vi "_Update Oscillators.vi"(4 "Pole In":bool[](array[boolean]), 5 "UpdateInput (F)":bool, 6 "ADC Array":i32[](array[numeric]), 7 "ADC Table":T1[](array[typedef]), 8 "Pole Swap (T)":bool=TRUE, 9 "Update (T)":bool=TRUE, 10 "Mode(pos)":bool=TRUE, 11 "Oscillator Settings":refnum<vi>) -> (1 "Q1RF Frequency":dbl, 2 "Instrument":string[](array[string]), 3 "Pole":bool[](array[boolean]))   [LabVIEW 2018]
uses:
  Type/_RT Configuration 2.ctl
  Type/_RT Command.ctl
  Configuration/_Global Configuration.vi
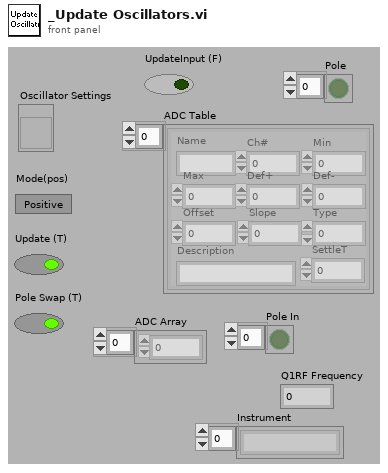
[diagram p1: front panel]
types:
  T1 = typedef "_RT Configuration 2.ctl" = cluster{"Name":string, "Ch#":u8, "Min":dbl, "Max":dbl, "Def+":dbl, "Def-":dbl, "Offset":dbl, "Slope":dbl, "Type":u8, "Description":string, "SettleT":dbl}
  T2 = typedef "_RT Instrument 2.ctl" = cluster{"Table":T1[], "Instrument":string[]}
  T3 = typedef "_RT Command.ctl" = enum16{"xml Start Run", "xml Start Actual Run", "xml Stop Run", "xml Runtime Update", "xml Get Status", "xml Get Table", "xml Set Table", "xml Get Configuration", "xml System Status", "xml Set LC Input Logic", "xml Get Data", "xml Get Info", "Start", "StartActualRun", "Stop", "Runtime Update", "Get Data", "Get Info", "Get Status", "Get Param", "Get Config", "Get Table", "Read ADC", "Set Oscillator", "Update Config", "Update Table", "Set All Pol", "Set Pol and DC", "Set Max Mass", "Toggle RP", "Toggle EL", "Set PIC", "Initialize Turbo", "Send Turbo Comm", "Close Turbo", "P1", "P2", "P3", "Send Serial", "Set LC Out", "Get LC In", "Read VAC", "Test Table", "Toggle Power", "Get Startup", "Set Startup", "Get ADC Table", "Set ADC Table", "Get Brief Status", "Get Detail Status", "Auxiliary Update", "Set CC Logics", "Test Channel", "Set CC Input Logics", "Ignore Error", "invalid"}
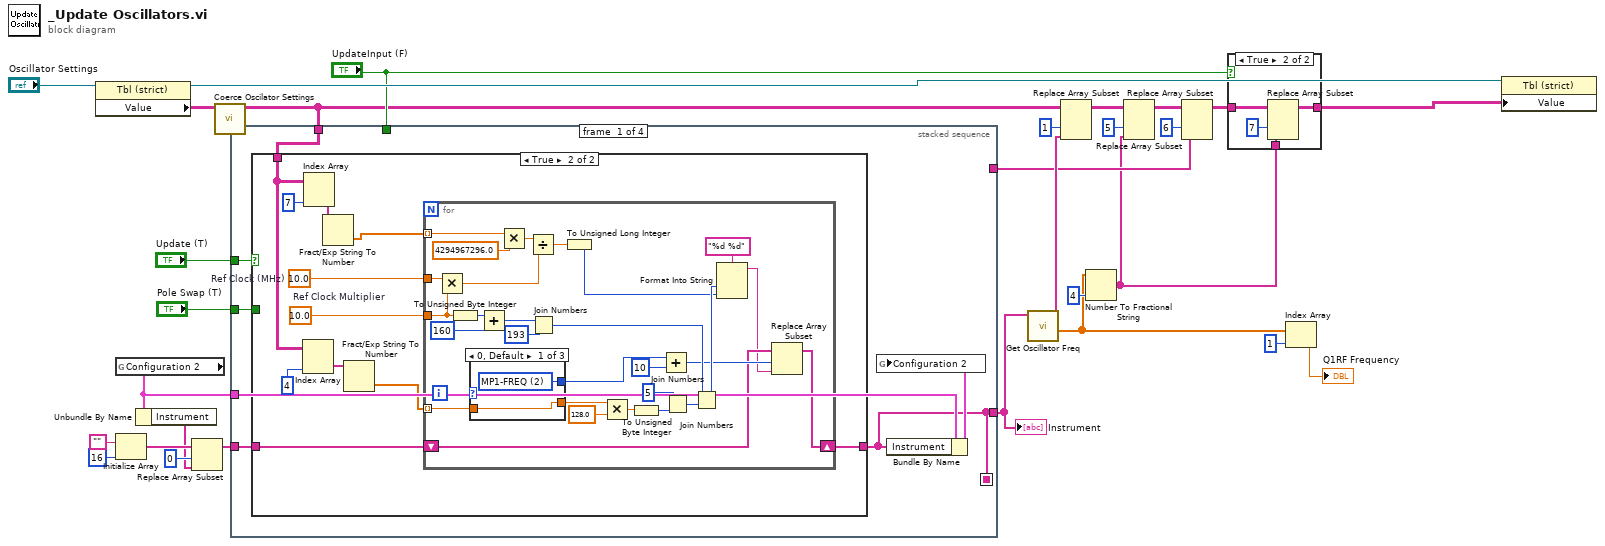
[diagram p0: block diagram]
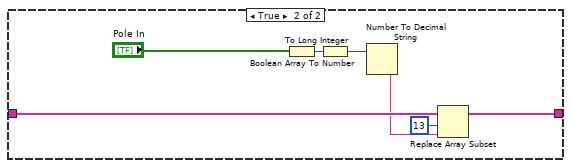
[diagram p4: hidden frame]
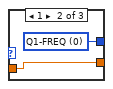
[diagram p5: hidden frame]
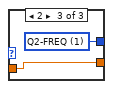
[diagram p6: hidden frame]
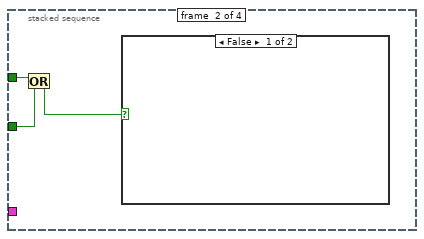
[diagram p7: hidden frame]
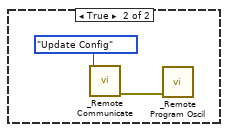
[diagram p8: hidden frame]
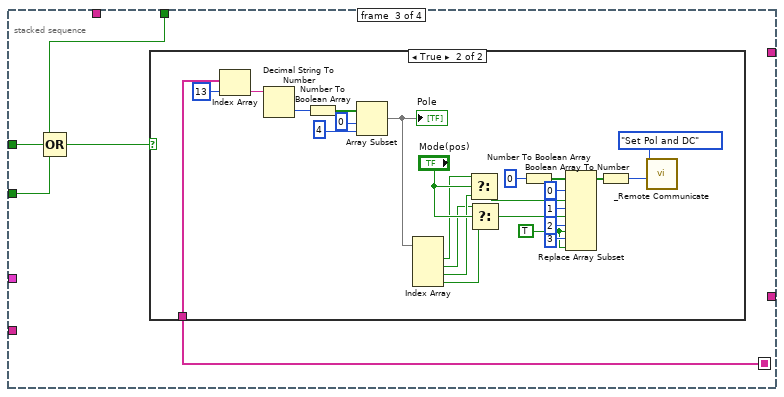
[diagram p9: hidden frame]
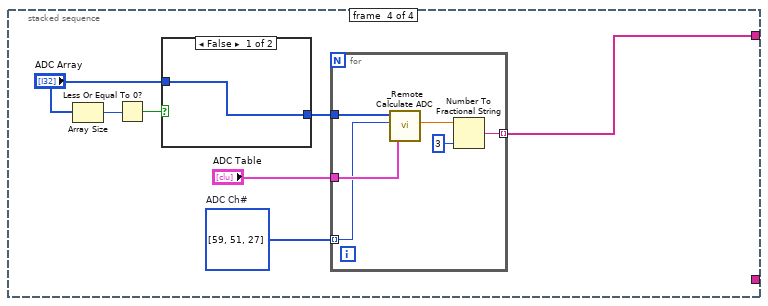
[diagram p11: hidden frame]
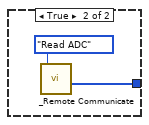
[diagram p12: hidden frame]
diagram:
  n1 = property class="Tbl (strict)"(reference="Oscillator Settings") -> (reference out=w21:refnum<vi>, "Value"=w14:string[][])  [unwired: 1 in, 1 out]
  n2 = global read "_Global Configuration.vi" "Configuration 2"() -> (w22:T2)
  n3 = Initialize Array("", 16 ("dimension size")) -> (w26:string[])
  n4 = Unbundle By Name(w22) -> ("Instrument"=w24:string[])
  n5 = Replace Array Subset(array=w26, new element=w24, index=0) -> (w23:string[])
  n6 = call "Coerce Oscilator Settings.vi"("Oscillator Settings in"=w14) -> ("Oscillator Settings out"=w4:string[][])  [unwired: 10 in]
  n7 = stacked-sequence {
    seq-local: [w30 _ _ _] -> [_ _ w103 _]
    tunnel: w4 -> [w36 _ _ _]
    tunnel: w23 -> [w35 _ _ _]
    tunnel: w22 -> [w33 _ _ _]
    tunnel: [w30 _ _ _] -> w16
    tunnel: "Update (T)" -> [w32 w96 w101 _]
    tunnel: "Pole Swap (T)" -> [w31 w95 w100 _]
    tunnel: [_ _ _ w132] -> w8
    tunnel: "UpdateInput (F)" -> [_ _ w102 _]
    frame #0 {
      n8 = case shown="True" w32 {
        tunnel: w36 -> [_ w51]
        tunnel: w35 -> [w39 w53]
        tunnel: [w37 w52] -> w30
        tunnel: w31 -> [w38 _]
        frame False {
          n9 = case shown="False" w38 {
            tunnel: w39 -> [w40 w45]
            tunnel: [w40 w44] -> w37
            frame False {
            }
            frame True {
              n10 = Boolean Array To Number(Boolean array="Pole In") -> (number=w46:u32)
              n11 = To Long Integer(number=w46) -> (32bit integer=w47:i32)
              n12 = Number To Decimal String(number=w47) -> (decimal integer string=w43:string)  [unwired: 1 out]
              n13 = Replace Array Subset(array=w45, new element=w43, index=13) -> (w44:string[])
            }
          }
        }
        frame True {
          w55 = 10.0  # Ref Clock Multiplier
          w56 = 10.0  # Ref Clock (MHz)
          n14 = Index Array(array=w51, index (col)=4 ("disabled index (col)")) -> (element=w50:string[])  [unwired: 1 in]
          n15 = Index Array(array=w51, index (col)=7 ("disabled index (col)")) -> (element=w57:string[])  [unwired: 1 in]
          n16 = Fract/Exp String To Number(string=w57) -> (number=w54:dbl[])  [unwired: 4 out]
          n17 = Fract/Exp String To Number(string=w50) -> (number=w48:dbl[])  [unwired: 4 out]
          n18 = for {
            tunnel: w56 -> [w83]
            tunnel: w55 -> [w80]
            tunnel: w54 -> [w61] mode=indexing
            shift-right: [w62] -> w52
            shift-left: w53 -> [w64]
            tunnel: w48 -> [w59] mode=indexing
            i -> [w87]
            n19 = Multiply(x=w83, y=w80) -> (x*y=w82:dbl)
            n20 = To Unsigned Byte Integer(number=w80) -> (unsigned 8bit integer=w81:u8)
            n21 = case shown="0, Default" w87 {
              tunnel: [w89 w91 w93] -> w66
              tunnel: w59 -> [w88 w90 w92]
              tunnel: [w88 w90 w92] -> w60
              frame 0, Default {
                w89 = u32 2 items=["Q1-FREQ", "Q2-FREQ", "MP1-FREQ"] ("Chip Select")
              }
              frame 1 {
                w91 = u32 0 items=["Q1-FREQ", "Q2-FREQ", "MP1-FREQ"] ("Chip Select")
              }
              frame 2 {
                w93 = u32 1 items=["Q1-FREQ", "Q2-FREQ", "MP1-FREQ"] ("Chip Select")
              }
            }
            n22 = Add(x=w81, y=u8 160) -> (x+y=w78:u8)
            n23 = Multiply(x=w61, y=4294967296.0) -> (x*y=w86:dbl)
            n24 = Divide(x=w86, y=w82) -> (x/y=w85:dbl)
            n25 = Join Numbers(hi=w78, lo=u8 193 ("Register 1")) -> ((hi.lo)=w71:u16)
            n26 = To Unsigned Long Integer(number=w85) -> (unsigned 32bit integer=w68:u32)
            n27 = Multiply(x=w60, y=128.0) -> (x*y=w75:dbl)
            n28 = To Unsigned Byte Integer(number=w75) -> (unsigned 8bit integer=w74:u8)
            n29 = Add(x=w66, y=u32 10) -> (x+y=w65:u32)
            n30 = Join Numbers(hi=u8 5 ("Register 6"), lo=w74) -> ((hi.lo)=w72:u16)
            n31 = Join Numbers(hi=w71, lo=w72) -> ((hi.lo)=w69:u32)
            n32 = Format Into String(format string="%d %d", w69, w68) -> (resulting string=w63:string)  [unwired: 2 in, 1 out]
            n33 = Replace Array Subset(array=w64, new element=w63, index=w65) -> (w62:string[])
          }
        }
      }
      n34 = Bundle By Name(cluster=w33, "Instrument"=w30) -> (w34:T2)
      n35 = global write "_Global Configuration.vi" "Configuration 2"(w34) -> ()
    }
    frame #1 {
      n36 = Or(x=w96, y=w95) -> (x .or. y?=w94:bool)
      n37 = case shown="False" w94 {
        frame False {
        }
        frame True {
          n38 = call "_Remote Communicate.vi"("Command"=_RT_Command."Update Config") -> ("error out"=w97:errorcluster)  [unwired: 5 in, 3 out]
          n39 = call "_Remote Program Oscil.vi"("error in (no error)"=w97) -> ()  [unwired: 1 out]
        }
      }
    }
    frame #2 {
      n40 = Compound Arithmetic op=OR(w102, w101, w100) -> (w99:bool)
      n41 = case shown="True" w99 {
        tunnel: w103 -> [_ w122]
        frame False {
        }
        frame True {
          w114 = TRUE ("new element/subarray")
          n42 = Index Array(array=w122, index=13) -> (element=w124:string)
          n43 = Decimal String To Number(string=w124) -> (number=w125:i32)  [unwired: 3 out]
          n44 = Number To Boolean Array(number=w125) -> (Boolean array=w126:bool[])
          n45 = Array Subset(array=w126, index=0, length=4) -> (w104:bool[])
          "Pole" <- w104
          n46 = Index Array(array=w104) -> (element #1=w110:bool, element #2=w106:bool, element #3=w109:bool, element #4=w108:bool)  [unwired: 4 in]
          n47 = Select(t=w110, s="Mode(pos)", f=w109) -> (s? t:f=w107:bool)
          n48 = Select(t=w106, s="Mode(pos)", f=w108) -> (s? t:f=w105:bool)
          n49 = Number To Boolean Array(number=u16 0) -> (Boolean array=w116:bool[])
          n50 = Replace Array Subset(array=w116, new element #1=w107, index #1=0 ("index"), new element #2=w105, index #2=1 ("index"), new element #3=w114, index #3=2 ("index"), new element #4=w114, index #4=3 ("index")) -> (w121:bool[])
          n51 = Boolean Array To Number(Boolean array=w121) -> (number=w112:u16)
          n52 = call "_Remote Communicate.vi"("DC Param"=w112, "Command"=_RT_Command."Set Pol and DC") -> ()  [unwired: 4 in, 4 out]
        }
      }
    }
    frame #3 {
      w135 = u8[] [59, 51, 27]  # ADC Ch#
      n53 = Array Size(array="ADC Array") -> (size(s)=w131:i32)
      n54 = Less Or Equal To 0?(x=w131) -> (x <= 0?=w130:bool)
      n55 = case shown="False" w130 {
        tunnel: [w136 w137] -> w134
        tunnel: "ADC Array" -> [w136 _]
        frame False {
        }
        frame True {
          n56 = call "_Remote Communicate.vi"("Command"=_RT_Command."Read ADC") -> ("Data Array"=w137:i32[])  [unwired: 5 in, 3 out]
        }
      }
      n57 = for {
        tunnel: w135 -> [w142] mode=indexing
        tunnel: w134 -> [w143]
        tunnel: "ADC Table" -> [w144]
        tunnel: [w139] -> w132 mode=indexing
        n58 = call "_Remote Calculate ADC.vi"("ADC Table"=w144, "ADC Channel (64)"=w142, "ADC Values"=w143) -> ("User Value"=w140:dbl)  [unwired: 1 in, 3 out]
        n59 = Number To Fractional String(number=w140, precision (6)=i16 3) -> (F-format string=w139:string)  [unwired: 2 out]
      }
    }
  }
  "Instrument" <- w16
  n60 = call "Get Oscillator Freq.vi"("Array 3"=w16) -> ("Oscillator Freqs"=w2:dbl[], "Tuning Word"=w12:string[])  [unwired: 7 in, 2 out]
  n61 = Replace Array Subset(array=w4, new element=w12, index (col)=1 ("disabled index (col)")) -> (w13:string[][])  [unwired: 1 in]
  n62 = Number To Fractional String(number=w2, precision (6)=i16 4) -> (F-format string=w1:string[])  [unwired: 2 out]
  n63 = Replace Array Subset(array=w13, new element=w1, index (col)=5 ("disabled index (col)")) -> (w10:string[][])  [unwired: 1 in]
  n64 = Replace Array Subset(array=w10, new element=w8, index (col)=6 ("disabled index (col)")) -> (w9:string[][])  [unwired: 1 in]
  n65 = case shown="True" "UpdateInput (F)" {
    tunnel: w1 -> [_ w148]
    tunnel: [w145 w147] -> w19
    tunnel: w9 -> [w145 w146]
    frame False {
    }
    frame True {
      n66 = Replace Array Subset(array=w146, new element=w148, index (col)=7 ("disabled index (col)")) -> (w147:string[][])  [unwired: 1 in]
    }
  }
  n67 = Index Array(array=w2, index=1) -> (element=→"Q1RF Frequency":dbl)
  n68 = property class="Tbl (strict)"(reference=w21, "Value"=w19) -> ()  [unwired: 1 in, 2 out]
